vi "MPS TX String.vi"(10 "Command":string, 11 "Header":string) -> (3 "TX Out":string)   [LabVIEW 2025]
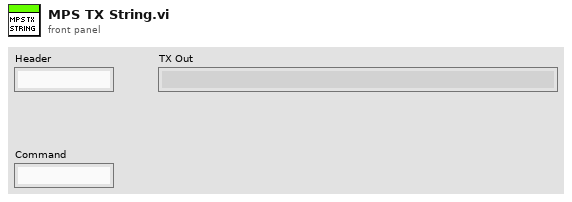
[diagram p1: front panel]
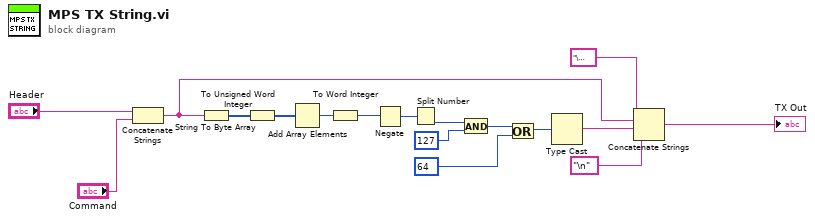
[diagram p0: block diagram]
diagram:
  n1 = Concatenate Strings("Header", "Command") -> (w14:string)
  n2 = String To Byte Array(string=w14) -> (unsigned byte array=w3:u8[])
  n3 = To Unsigned Word Integer(number=w3) -> (unsigned 16bit integer=w4:u16[])
  n4 = Add Array Elements(numeric array=w4) -> (sum=w5:u16)
  n5 = To Word Integer(number=w5) -> (16bit integer=w6:i16)
  n6 = Negate(x=w6) -> (-x=w7:i16)
  n7 = Split Number(x=w7) -> (lo(x)=w8:u8)  [unwired: 1 out]
  n8 = And(x=w8, y=u8 127) -> (x .and. y?=w10:u8)
  n9 = Or(x=w10, y=u8 64) -> (x .or. y?=w12:u8)
  n10 = Type Cast(x=w12) -> (*(type *) &x=w13:string)  [unwired: 1 in]
  n11 = Concatenate Strings("\u0002", w14, w13, "\n") -> (→"TX Out":string)
